vi "Format ModAcc.vi"(10 "Modulation Results":T1) -> (2 "Modulation Results":T2)   [LabVIEW 2015, in "niDTS BT.lvlib" / "niDTS BT INSTR TX.lvclass"]
uses:
  niDTS BT INSTR TX.lvclass
  Includes/niDTS BT INSTR TX INC ModAcc Result.ctl
  Tests/Tx Test/Includes/niDTS BT Tx Test INC DEVM Results.ctl
  Tests/Tx Test/Includes/niDTS BT Tx Test INC CF Stability Results.ctl
  Tests/Tx Test/Includes/niDTS BT Tx Test INC CFO Resutls.ctl
  Tests/Tx Test/Includes/niDTS BT Tx Test INC Character Results.ctl
  niDTS BT.lvlib
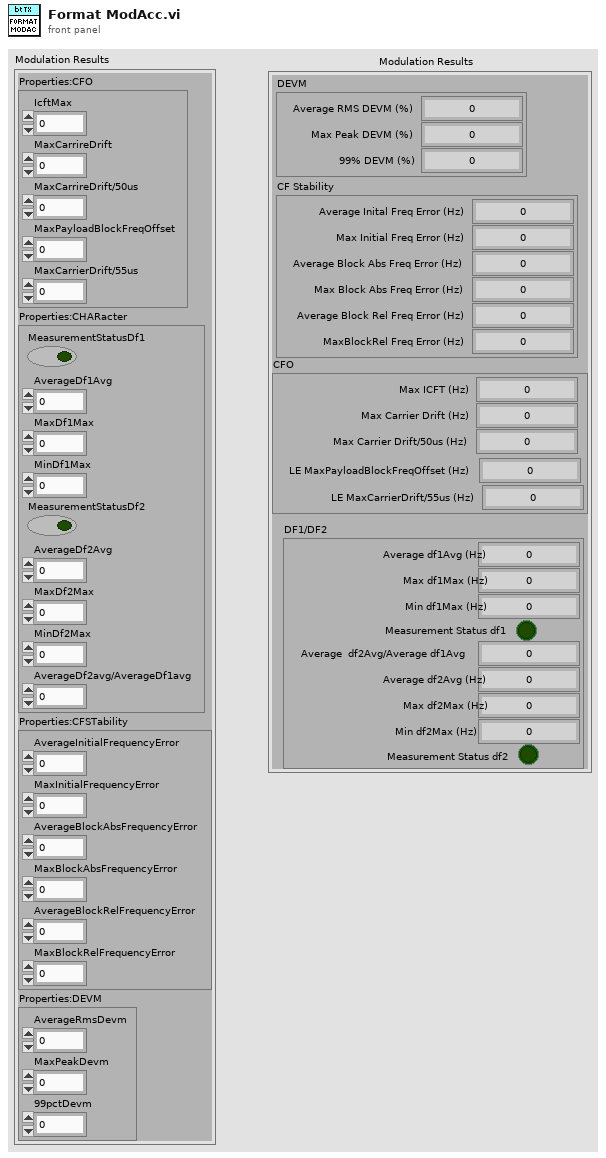
[diagram p1: front panel]
types:
  T1 = cluster{"Properties:CFO":cluster{"IcftMax":dbl, "MaxCarrireDrift":dbl, "MaxCarrireDrift/50us":dbl, "MaxPayloadBlockFreqOffset":dbl, "MaxCarrierDrift/55us":dbl}, "Properties:CHARacter":cluster{"MeasurementStatusDf1":bool, "AverageDf1Avg":dbl, "MaxDf1Max":dbl, "MinDf1Max":dbl, "MeasurementStatusDf2":bool, "AverageDf2Avg":dbl, "MaxDf2Max":dbl, "MinDf2Max":dbl, "AverageDf2avg/AverageDf1avg":dbl}, "Properties:CFSTability":cluster{"AverageInitialFrequencyError":dbl, "MaxInitialFrequencyError":dbl, "AverageBlockAbsFrequencyError":dbl, "MaxBlockAbsFrequencyError":dbl, "AverageBlockRelFrequencyError":dbl, "MaxBlockRelFrequencyError":dbl}, "Properties:DEVM":cluster{"AverageRmsDevm":dbl, "MaxPeakDevm":dbl, "99pctDevm":dbl}}
  T2 = typedef "niDTS BT.lvlib/niDTS BT INSTR TX.lvclass/niDTS BT INSTR TX INC ModAcc Result.ctl" = cluster{"DEVM":T3, "CF Stability":T4, "CFO":T5, "DF1/DF2":T6}
  T3 = typedef "niDTS BT.lvlib/niDTS BT Tx Test INC DEVM Results.ctl" = cluster{"Average RMS DEVM (%)":dbl, "Max Peak DEVM (%)":dbl, "99% DEVM (%)":dbl}
  T4 = typedef "niDTS BT.lvlib/niDTS BT Tx Test INC CF Stability Results.ctl" = cluster{"Average Inital Freq Error (Hz)":dbl, "Max Initial Freq Error (Hz)":dbl, "Average Block Abs Freq Error (Hz)":dbl, "Max Block Abs Freq Error (Hz)":dbl, "Average Block Rel Freq Error (Hz)":dbl, "MaxBlockRel Freq Error (Hz)":dbl}
  T5 = typedef "niDTS BT.lvlib/niDTS BT Tx Test INC CFO Resutls.ctl" = cluster{"Max ICFT (Hz)":dbl, "Max Carrier Drift (Hz)":dbl, "Max Carrier Drift/50us (Hz)":dbl, "LE MaxPayloadBlockFreqOffset (Hz)":dbl, "LE MaxCarrierDrift/55us (Hz)":dbl}
  T6 = typedef "niDTS BT.lvlib/niDTS BT Tx Test INC Character Results.ctl" = cluster{"Average df1Avg (Hz)":dbl, "Max df1Max (Hz)":dbl, "Min df1Max (Hz)":dbl, "Measurement Status df1":bool, "Average  df2Avg/Average df1Avg":dbl, "Average df2Avg (Hz)":dbl, "Max df2Max (Hz)":dbl, "Min df2Max (Hz)":dbl, "Measurement Status df2":bool}
  T7 = cluster{"AverageRmsDevm":dbl, "MaxPeakDevm":dbl, "99pctDevm":dbl}
  T8 = cluster{"AverageInitialFrequencyError":dbl, "MaxInitialFrequencyError":dbl, "AverageBlockAbsFrequencyError":dbl, "MaxBlockAbsFrequencyError":dbl, "AverageBlockRelFrequencyError":dbl, "MaxBlockRelFrequencyError":dbl}
  T9 = cluster{"IcftMax":dbl, "MaxCarrireDrift":dbl, "MaxCarrireDrift/50us":dbl, "MaxPayloadBlockFreqOffset":dbl, "MaxCarrierDrift/55us":dbl}
  T10 = cluster{"MeasurementStatusDf1":bool, "AverageDf1Avg":dbl, "MaxDf1Max":dbl, "MinDf1Max":dbl, "MeasurementStatusDf2":bool, "AverageDf2Avg":dbl, "MaxDf2Max":dbl, "MinDf2Max":dbl, "AverageDf2avg/AverageDf1avg":dbl}
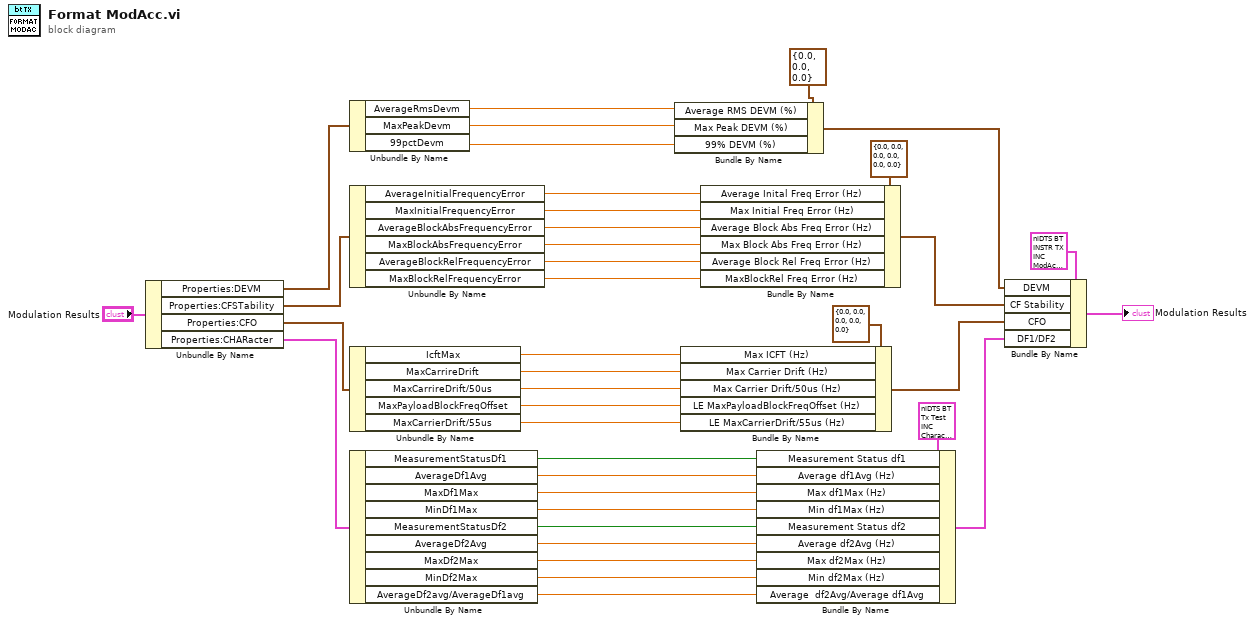
[diagram p0: block diagram]
diagram:
  n1 = Unbundle By Name("Modulation Results") -> ("Properties:DEVM"=w37:T7, "Properties:CFSTability"=w22:T8, "Properties:CFO"=w23:T9, "Properties:CHARacter"=w30:T10)
  n2 = Unbundle By Name(w37) -> ("AverageRmsDevm"=w35:dbl, "MaxPeakDevm"=w33:dbl, "99pctDevm"=w32:dbl)
  n3 = Unbundle By Name(w22) -> ("AverageInitialFrequencyError"=w16:dbl, "MaxInitialFrequencyError"=w15:dbl, "AverageBlockAbsFrequencyError"=w14:dbl, "MaxBlockAbsFrequencyError"=w13:dbl, "AverageBlockRelFrequencyError"=w12:dbl, "MaxBlockRelFrequencyError"=w11:dbl)
  n4 = Unbundle By Name(w23) -> ("IcftMax"=w19:dbl, "MaxCarrireDrift"=w18:dbl, "MaxCarrireDrift/50us"=w17:dbl, "MaxPayloadBlockFreqOffset"=w5:dbl, "MaxCarrierDrift/55us"=w4:dbl)
  n5 = Unbundle By Name(w30) -> ("MeasurementStatusDf1"=w3:bool, "AverageDf1Avg"=w29:dbl, "MaxDf1Max"=w28:dbl, "MinDf1Max"=w27:dbl, "MeasurementStatusDf2"=w2:bool, "AverageDf2Avg"=w26:dbl, "MaxDf2Max"=w25:dbl, "MinDf2Max"=w24:dbl, "AverageDf2avg/AverageDf1avg"=w1:dbl)
  n6 = Bundle By Name(cluster=T3 {"Average RMS DEVM (%)"=0.0, "Max Peak DEVM (%)"=0.0, "99% DEVM (%)"=0.0} ("DEVM"), "Average RMS DEVM (%)"=w35, "Max Peak DEVM (%)"=w33, "99% DEVM (%)"=w32) -> (w34:T3)
  n7 = Bundle By Name(cluster=T5 {"Max ICFT (Hz)"=0.0, "Max Carrier Drift (Hz)"=0.0, "Max Carrier Drift/50us (Hz)"=0.0, "LE MaxPayloadBlockFreqOffset (Hz)"=0.0, "LE MaxCarrierDrift/55us (Hz)"=0.0} ("CFO"), "Max ICFT (Hz)"=w19, "Max Carrier Drift (Hz)"=w18, "Max Carrier Drift/50us (Hz)"=w17, "LE MaxPayloadBlockFreqOffset (Hz)"=w5, "LE MaxCarrierDrift/55us (Hz)"=w4) -> (w9:T5)
  n8 = Bundle By Name(cluster=T4 {"Average Inital Freq Error (Hz)"=0.0, "Max Initial Freq Error (Hz)"=0.0, "Average Block Abs Freq Error (Hz)"=0.0, "Max Block Abs Freq Error (Hz)"=0.0, "Average Block Rel Freq Error (Hz)"=0.0, "MaxBlockRel Freq Error (Hz)"=0.0} ("CF Stability"), "Average Inital Freq Error (Hz)"=w16, "Max Initial Freq Error (Hz)"=w15, "Average Block Abs Freq Error (Hz)"=w14, "Max Block Abs Freq Error (Hz)"=w13, "Average Block Rel Freq Error (Hz)"=w12, "MaxBlockRel Freq Error (Hz)"=w11) -> (w10:T4)
  n9 = Bundle By Name(cluster=T6 {"Average df1Avg (Hz)"=0.0, "Max df1Max (Hz)"=0.0, "Min df1Max (Hz)"=0.0, "Measurement Status df1"=FALSE, "Average  df2Avg/Average df1Avg"=0.0, "Average df2Avg (Hz)"=0.0, "Max df2Max (Hz)"=0.0, "Min df2Max (Hz)"=0.0, "Measurement Status df2"=FALSE} ("DF1/DF2"), "Measurement Status df1"=w3, "Average df1Avg (Hz)"=w29, "Max df1Max (Hz)"=w28, "Min df1Max (Hz)"=w27, "Measurement Status df2"=w2, "Average df2Avg (Hz)"=w26, "Max df2Max (Hz)"=w25, "Min df2Max (Hz)"=w24, "Average  df2Avg/Average df1Avg"=w1) -> (w31:T6)
  n10 = Bundle By Name(cluster=T2 {"DEVM"={"Average RMS DEVM (%)"=0.0, "Max Peak DEVM (%)"=0.0, "99% DEVM (%)"=0.0}, "CF Stability"={"Average Inital Freq Error (Hz)"=0.0, "Max Initial Freq Error (Hz)"=0.0, "Average Block Abs Freq Error (Hz)"=0.0, "Max Block Abs Freq Error (Hz)"=0.0, "Average Block Rel Freq Error (Hz)"=0.0, "MaxBlockRel Freq Error (Hz)"=0.0}, "CFO"={"Max ICFT (Hz)"=0.0, "Max Carrier Drift (Hz)"=0.0, "Max Carrier Drift/50us (Hz)"=0.0, "LE MaxPayloadBlockFreqOffset (Hz)"=0.0, "LE MaxCarrierDrift/55us (Hz)"=0.0}, "DF1/DF2"={"Average df1Avg (Hz)"=0.0, "Max df1Max (Hz)"=0.0, "Min df1Max (Hz)"=0.0, "Measurement Status df1"=FALSE, "Average  df2Avg/Average df1Avg"=0.0, "Average df2Avg (Hz)"=0.0, "Max df2Max (Hz)"=0.0, "Min df2Max (Hz)"=0.0, "Measurement Status df2"=FALSE}} ("output cluster"), "DEVM"=w34, "CF Stability"=w10, "CFO"=w9, "DF1/DF2"=w31) -> (→"Modulation Results":T2)
